vi "stringConvertToDate2_yyyymmdd.vi"(1 "input_str_yyyymmdd":string="2015/11/23 8:14:18") -> (0 "show_date":timestamp)   [LabVIEW 2011]
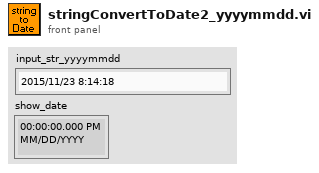
[diagram p1: front panel]
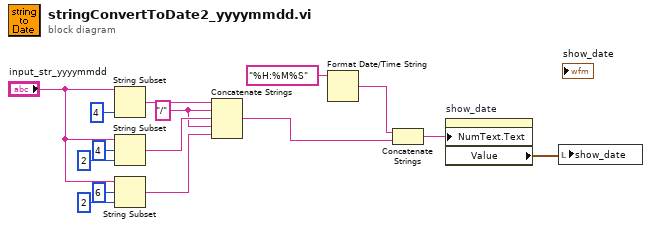
[diagram p0: block diagram]
diagram:
  w5 = "/" ("字符串")
  n1 = String Subset(string="input_str_yyyymmdd", length (rest)=4 ("长度（剩余）")) -> (substring=w7:string)  [unwired: 1 in]
  n2 = String Subset(string="input_str_yyyymmdd", offset (0)=4 ("偏移量(0)"), length (rest)=2 ("长度（剩余）")) -> (substring=w6:string)
  n3 = String Subset(string="input_str_yyyymmdd", offset (0)=6 ("偏移量(0)"), length (rest)=2 ("长度（剩余）")) -> (substring=w4:string)
  n4 = Concatenate Strings(w7, w5, w6, w5, w4) -> (w3:string)
  n5 = Format Date/Time String(time format string (%c)="%H:%M%S" ("时间格式字符串(%c)")) -> (date/time string=w1:string)  [unwired: 2 in]
  n6 = Concatenate Strings(w1, w3) -> (w14:string)
  n7 = property on="show_date" class="AbsTime (严格)"("NumText.Text"=w14) -> ("Value"=w15:timestamp)  [unwired: 2 in, 2 out]
  n8 = local write "show_date"(w15) -> ()
